vi "VCP-Demo.vi"() -> ()   [LabVIEW 2021]
panel:
  in  "Read":T1={"Index"="``", "Sub-Index"="\u0000", "Data-Size (in Byte)"=1, FALSE} {"Data-Size (in Byte)" min=1 max=4 step=1 format="%x"}
  out "Answer":i32
  in  "Write":T2={"Data (dec)"=0, FALSE, "Index"="``", "Sub-Index"="\u0000", "Data-Size (in Byte)"=1} {"Data-Size (in Byte)" min=1 max=4 step=1 format="%x"; "Data (dec)" step=1}
  in  "?":bool
  out "error out":errorcluster
  in  "error in":errorcluster
  in  "ComPort":refnum<visa-resource-name>="COM1"
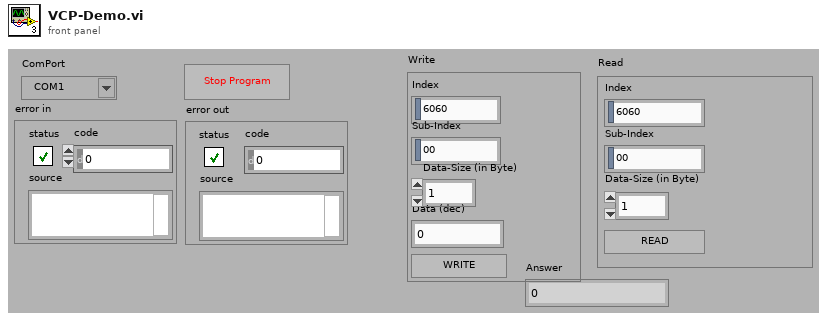
[diagram p1: front panel]
types:
  T1 = cluster{"Index":string, "Sub-Index":string, "Data-Size (in Byte)":u8, bool}
  T2 = cluster{"Data (dec)":i32, bool, "Index":string, "Sub-Index":string, "Data-Size (in Byte)":u8}
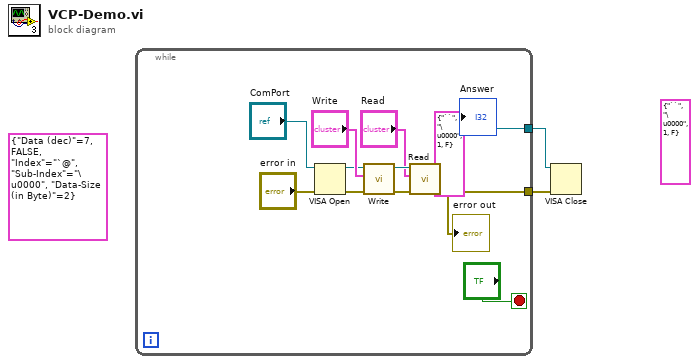
[diagram p0: block diagram]
diagram:
  (unwired) T2 {"Data (dec)"=7, FALSE, "Index"="`@", "Sub-Index"="\u0000", "Data-Size (in Byte)"=2} ("Write")
  (unwired) T1 {"Index"="``", "Sub-Index"="\u0000", "Data-Size (in Byte)"=1, FALSE} ("Read")
  n1 = while {
    tunnel: [w5] -> w2
    tunnel: [w7] -> w1
    stop <- "?" stop-if-true
    (unwired) T1 {"Index"="``", "Sub-Index"="\u0000", "Data-Size (in Byte)"=1, FALSE} ("Read")
    n2 = VISA Open(error in (no error)="error in", VISA resource name="ComPort") -> (VISA resource name=w9:refnum<visa-resource-name>, error out=w10:errorcluster)  [unwired: 3 in]
    n3 = call "Write.vi"("error in"=w10, "Write"="Write", "ComPort In"=w9) -> ("error out"=w6:errorcluster, "ComPort Out"=w8:refnum<visa-resource-name>)  [unwired: 7 in]
    n4 = call "Read.vi"("error out"=w6, "Read"="Read", "ComPort In"=w8) -> ("error out 2"=w5:errorcluster, "Answer"=→"Answer":i32, "ComPort Out"=w7:refnum<visa-resource-name>)  [unwired: 6 in]
    "error out" <- w5
  }
  n5 = VISA Close(VISA resource name=w1, error in (no error)=w2) -> ()  [unwired: 1 out]
